vi "flow-builder.ph-dosing.vi"(7 "Proc Name":string, 8 "error in":errorcluster, 9 "Unit Index":i32, 11 "Cluster":T3 {"ORP Dosing"."MIX Limit" format="%d [s]"; "ORP Dosing"."MIX Dose" format="%d [s]"; "PH Dosing"."ACID Limit" format="%d [s]"; "PH Dosing"."BASE Limit" format="%d [s]"; "PH Dosing"."ACID Dose" format="%d [s]"; "PH Dosing"."BASE Dose" format="%d [s]"; "EC Dosing"."BETA2 Limit" format="%d [s]"; "EC Dosing"."ALFA2 Limit" format="%d [s]"; "EC Dosing"."ALFA2 Dose" format="%d [s]"; "EC Dosing"."BETA2 Dose" format="%d [s]"; "EC Dosing"."BETA1 Limit" format="%d [s]"; "EC Dosing"."ALFA1 Limit" format="%d [s]"; "EC Dosing"."ALFA1 Dose" format="%d [s]"; "EC Dosing"."BETA1 Dose" format="%d [s]"; "Main"."DailyActivityHours"."Begin Time" format="ON:    %<%H:%M>T"; "Main"."DailyActivityHours"."End Time" format="OFF:    %<%H:%M>T"; "Main"."WashTimes"."Out" format="Wash out: %d [sec]"; "Main"."WashTimes"."In" format="Wash in: %d [sec]"; "Water Dosing"."Water Limit" format="%d [s]"; "Water Dosing"."Water Dose" format="%d [s]"}) -> (0 "error out":errorcluster, 1 "WillDose?":bool, 2 "status":string, 3 "Flow out":T1[](array[typedef]))   [LabVIEW 2024]
uses:
  controls/UiNutritionPanel.ctl
  controls/UiScheduleTimestamp.ctl
  controls/UiStepBuilder.ctl
  controls/type.step-builder.ctl
  controls/enum-ntr-io-format.ctl
  io.interface.serial.vi
  <vilib>/Utility/error.llb/Clear Errors.vi
  <vilib>/Utility/error.llb/Trim Whitespace One-Sided.vi
  Polymorphics/variantCtrlIo.vi
  globals/globals-engine.vi
  util.environment.vi
  util-address-parser.vi
  util-address-builder.vi
  util.DO.ToString.vi
  Polymorphics/io.command-builder.vi
  Polymorphics/io.command-builder.DO.vi
  Polymorphics/io.command-builder.AI.vi
  Polymorphics/io.command-builder.DI.vi
  io.frame.vi
  io.visa.vi
  io.responseValidator.vi
  Polymorphics/io.command-parser.DI.vi
  Polymorphics/io.command-parser.AI.vi
  step.util.flag-matching.vi
  util.file.record.vi
panel:
  out "Dosing Tabel":cluster{"Dose Time":dbl, "Input":string}[](array[cluster])
  in  "simulator":dbl=3.0
  out "High Range":bool
  out "Low Range":bool
  out "Low Alarm":bool
  out "High Alarm":bool
  # "Water"
  # "EC"
  # "PH"
  # "ORP"
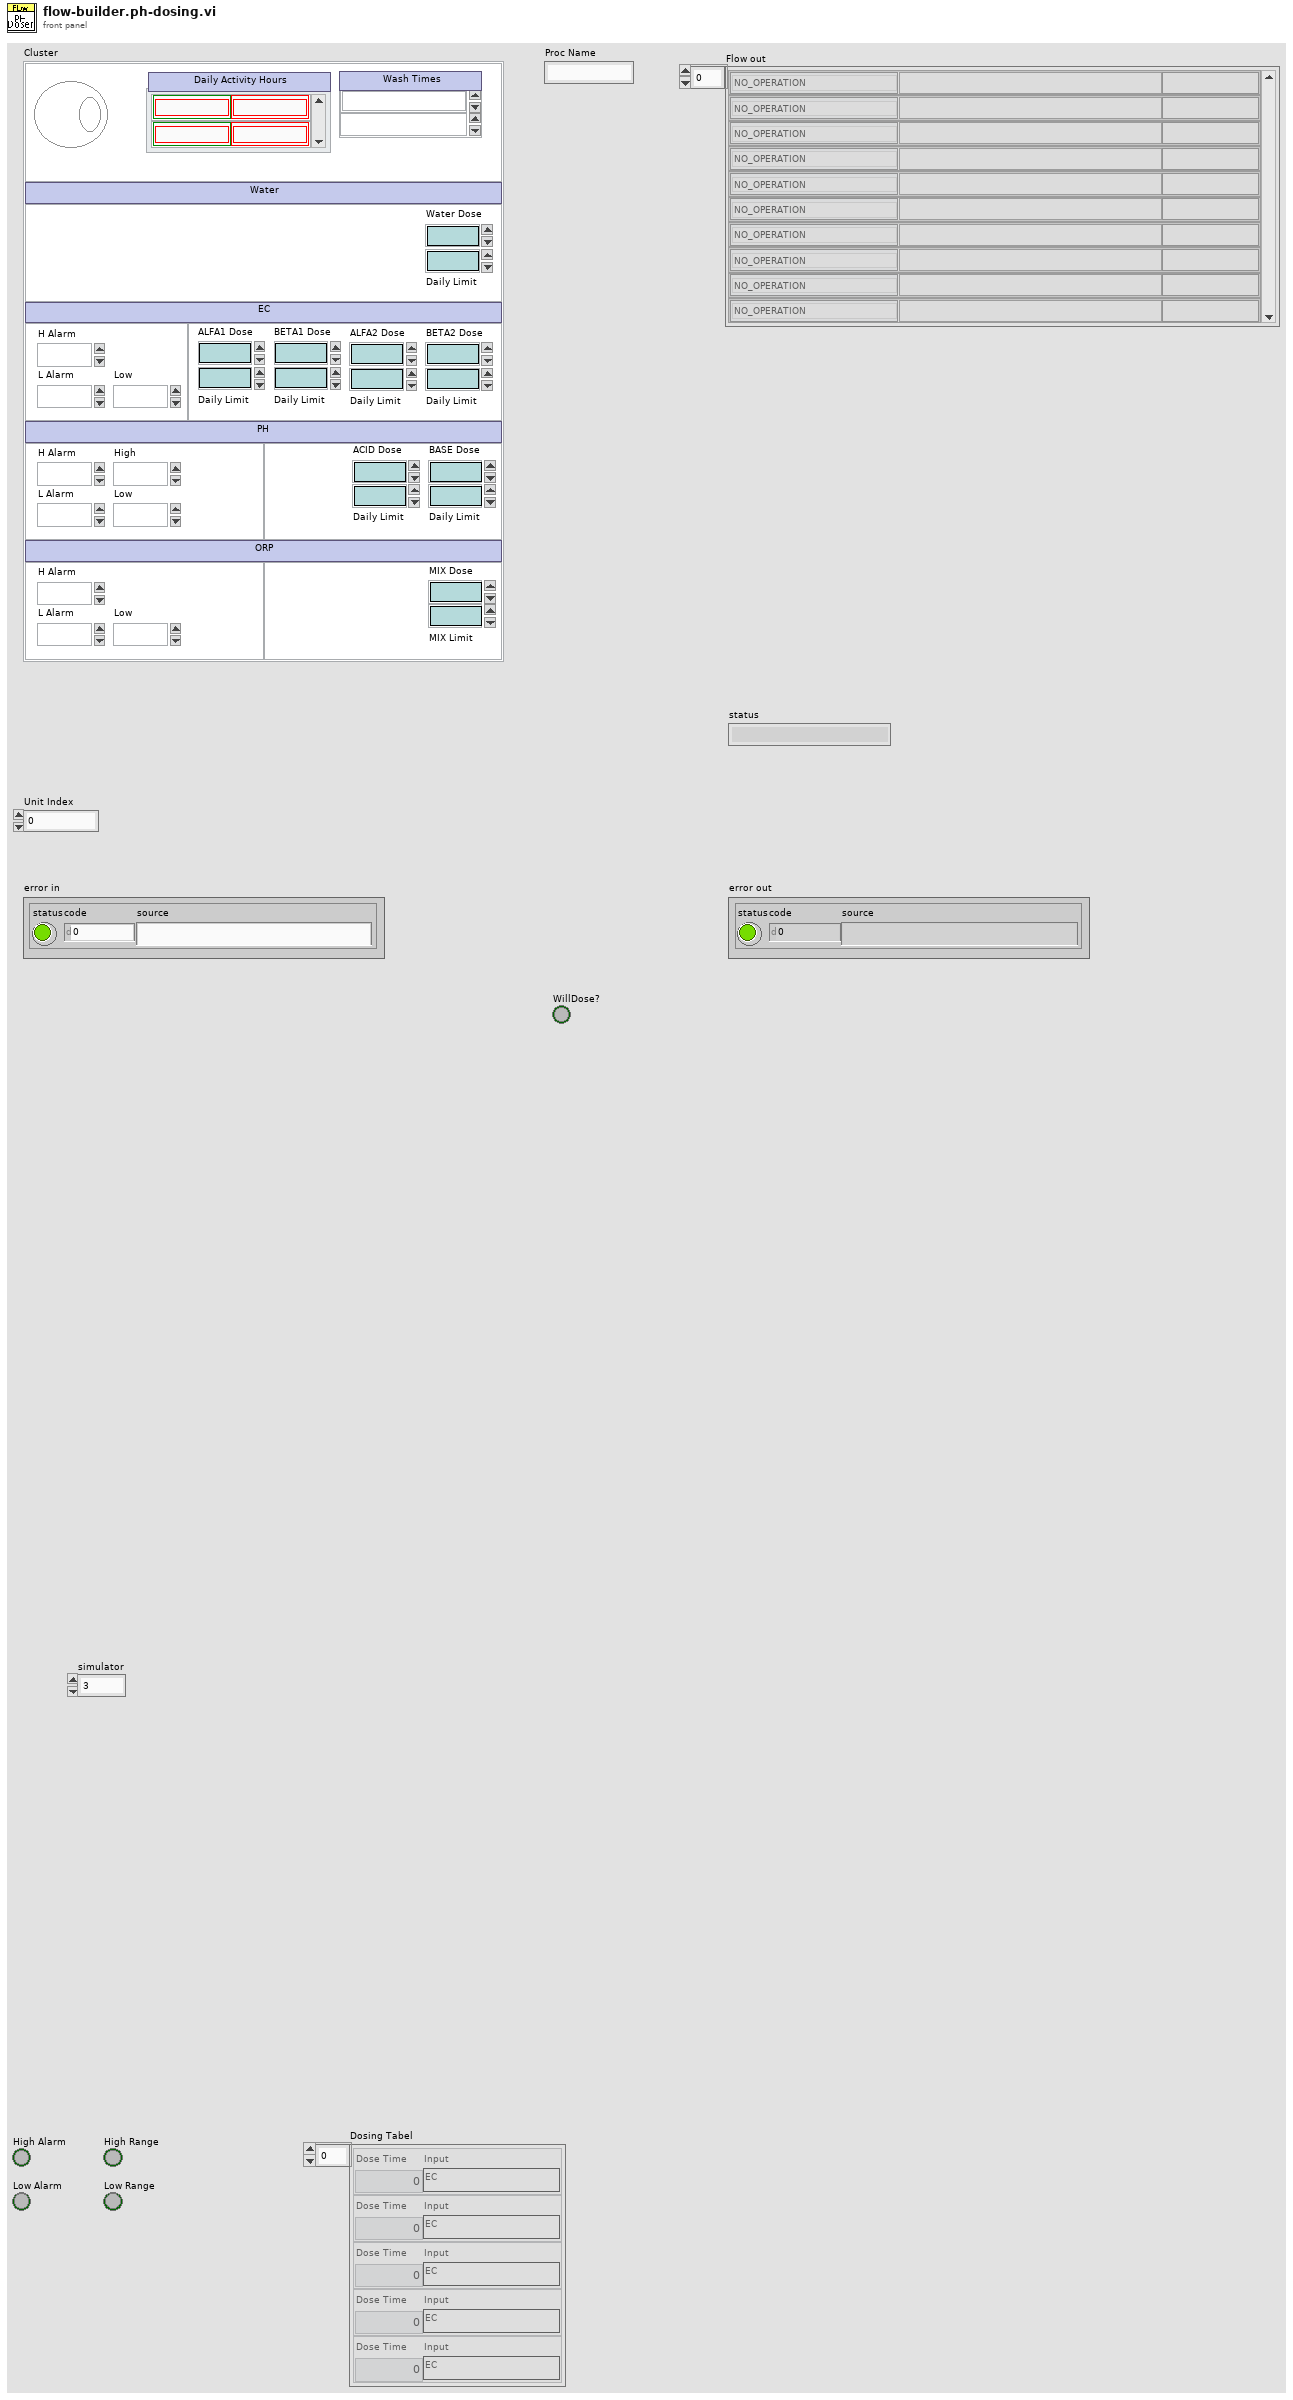
[diagram p1: front panel]
types:
  T1 = typedef "UiStepBuilder.ctl" = cluster{"Step Function":T2, "ParamString":string, "Step Label":string}
  T2 = typedef "type.step-builder.ctl" = enum16{"NO_OPERATION", "DELAY-JUMP", "DELAY", "JUMP", "COMPLETE", "SCHEDULER", "IRR-CHECK", "UNIT-CHECK", "UNIT-SAMPLE", "UNIT-DOSE", "LOG-REPORT", "LOG-MESSAGE", "IO-READ", "IO-READ-MANY", "IO-WRITE", "IO-COMPARE-OUT", "IO-COMPARE-IN", "PROC-START", "PROC-STOP", "PROC-LOAD", "PROC-IS-COMPLETED", "RECORD-MOVE", "GET-RH", "GET-UV", "GET-WD", "GET-WS", "OCS-CHECK", "OCS-RECORD"}
  T3 = typedef "UiNutritionPanel.ctl" = cluster{"Main":cluster{"Enable":bool, "WashTimes":cluster{"In":dbl, "Out":dbl}, "DailyActivityHours":cluster{"Begin Time":T4, "End Time":T4}[]}, "Water Dosing":cluster{"Water Dose":dbl, "Water Limit":dbl}, "EC Ranges":cluster{"H Alarm":dbl, "L Alarm":dbl, "Low":dbl}, "EC Dosing":cluster{"ALFA1 Dose":dbl, "ALFA1 Limit":dbl, "BETA1 Dose":dbl, "BETA1 Limit":dbl, "ALFA2 Dose":dbl, "ALFA2 Limit":dbl, "BETA2 Dose":dbl, "BETA2 Limit":dbl}, "PH Ranges":cluster{"H Alarm":dbl, "L Alarm":dbl, "High":dbl, "Low":dbl}, "PH Dosing":cluster{"ACID Dose":dbl, "ACID Limit":dbl, "BASE Dose":dbl, "BASE Limit":dbl}, "ORP Ranges":cluster{"H Alarm":dbl, "L Alarm":dbl, "Low":dbl}, "ORP Dosing":cluster{"MIX Dose":dbl, "MIX Limit":dbl}}
  T4 = typedef "UiScheduleTimestamp.ctl" = timestamp
  T5 = typedef "enum-ntr-io-format.ctl" = enum16{"UN_VLV%d", "UN_PMP%d", "UN_WL%d", "UN_PH", "UN_EC", "UN_ORP", "UN_WT", "UN_PH2", "UN_ALFA1", "UN_BETA1", "UN_ALFA2", "UN_BETA2", "UN_ACID", "UN_BASE", "UN_WATER", "UN_ORPMIX"}
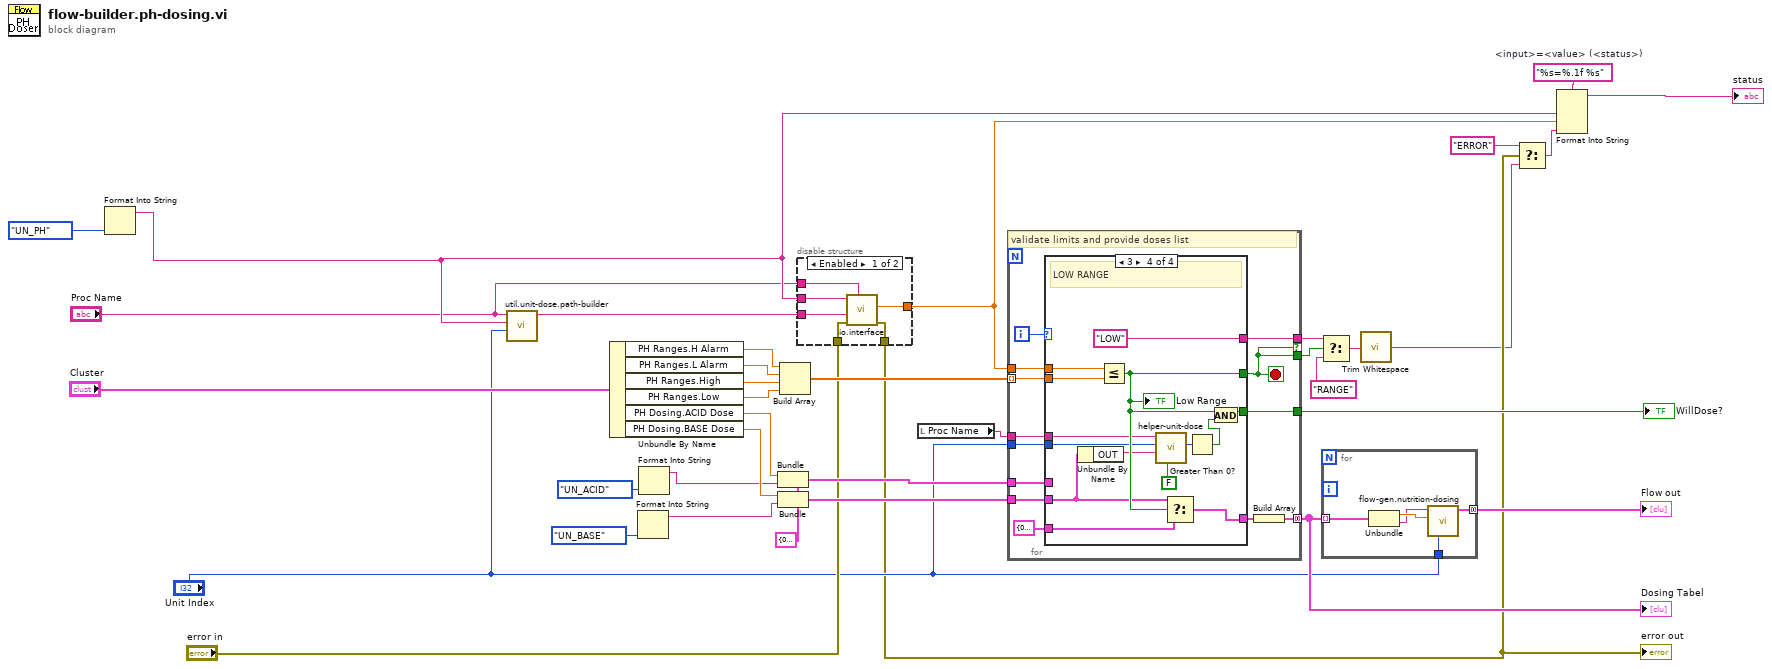
[diagram p0: block diagram]
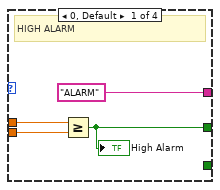
[diagram p2: hidden frame]
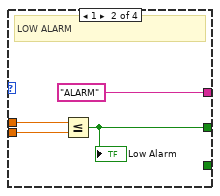
[diagram p3: hidden frame]
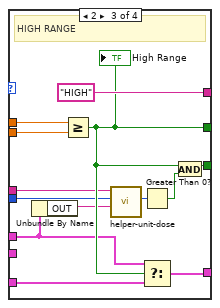
[diagram p4: hidden frame]
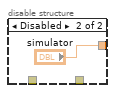
[diagram p5: hidden frame]
diagram:
  w5 = cluster{"ACID Dose":dbl, "OUT":string} {"ACID Dose"=0.0, "OUT"=""} ("cluster")
  w19 = "%s=%.1f %s"  # <input>=<value> (<status>)
  n1 = Format Into String(enum-ntr-io-format."UN_PH") -> (resulting string=w2:string)  [unwired: 3 in, 1 out]
  n2 = call "util.unit-dose.path-builder.vi"("Unit Index"="Unit Index", "Input"=w2, "Proc Name"="Proc Name") -> ("\\NUTRITION\\ORP\\ORP_U1_2024-08-16.*"=w14:string)  [unwired: 8 in]
  n3 = Unbundle By Name("Cluster") -> ("PH Ranges.H Alarm"=w36:dbl, "PH Ranges.L Alarm"=w34:dbl, "PH Ranges.High"=w33:dbl, "PH Ranges.Low"=w32:dbl, "PH Dosing.ACID Dose"=w28:dbl, "PH Dosing.BASE Dose"=w27:dbl)
  n4 = Format Into String(enum-ntr-io-format."UN_BASE") -> (resulting string=w6:string)  [unwired: 3 in, 1 out]
  n5 = Format Into String(enum-ntr-io-format."UN_ACID") -> (resulting string=w7:string)  [unwired: 3 in, 1 out]
  n6 = Bundle(cluster=w5, "ACID Dose"=w28, "OUT"=w7) -> (w26:cluster{"ACID Dose":dbl, "OUT":string})
  n7 = Bundle(cluster=w5, "ACID Dose"=w27, "OUT"=w6) -> (w25:cluster{"ACID Dose":dbl, "OUT":string})
  n8 = Build Array(w36, w34, w33, w32) -> (w35:dbl[])
  n9 = disable-structure shown="Enabled" {
    disable-tunnel: w2 -> [w42 _]
    disable-tunnel: [w41 "simulator"] -> w18
    disable-tunnel: [w40 _] -> w11
    disable-tunnel: "error in" -> [w39 _]
    disable-tunnel: w14 -> [w38 _]
    disable-tunnel: "Proc Name" -> [w37 _]
    frame Enabled {
      n10 = call "io.interface.vi"("Caller"=w37, "error in"=w39, "record filename.* (disabled if empty)"=w38, "IO Name in"=w42) -> ("error out"=w40:errorcluster, "Value out"=w41:dbl)  [unwired: 2 in, 4 out]
    }
    frame Disabled {
    }
  }
  "error out" <- w11
  n11 = local read "Proc Name"() -> (w15:string)
  n12 = for {
    tunnel: w35 -> [w55] mode=indexing
    tunnel: [w54] -> w21 if=w52
    tunnel: w18 -> [w53]
    tunnel: [w52] -> w22
    tunnel: [w49] -> w30 mode=concatenating
    tunnel: w26 -> [w48]
    tunnel: w25 -> [w50]
    tunnel: [w46] -> w16
    tunnel: "Unit Index" -> [w45]
    tunnel: w15 -> [w44]
    i -> [w56]
    stop <- w52 stop-if-true
    # "validate limits and provide doses list"
    n13 = case shown="3" w56 {
      tunnel: w55 -> [w59 w63 w76 w90]
      tunnel: [w57 w61 w72 w86] -> w52
      tunnel: ["ALARM" "ALARM" "HIGH" "LOW"] -> w54
      tunnel: w53 -> [w58 w62 w75 w89]
      tunnel: [_ _ w74 w88] -> w51
      tunnel: w50 -> [_ _ _ w83]
      tunnel: w48 -> [_ _ w65 _]
      tunnel: cluster{"BETA-2":dbl, "I/O":string} {"BETA-2"=0.0, "I/O"=""} ("f") -> [_ _ w73 w87]
      tunnel: [_ _ w67 w80] -> w46
      tunnel: w45 -> [_ _ w68 w81]
      tunnel: w44 -> [_ _ w69 w78]
      frame 0, Default {
        # "HIGH ALARM"
        n14 = Greater Or Equal?(x=w58, y=w59) -> (x >= y?=w57:bool)
        "High Alarm" <- w57
      }
      frame 1 {
        # "LOW ALARM"
        n15 = Less Or Equal?(x=w62, y=w63) -> (x <= y?=w61:bool)
        "Low Alarm" <- w61
      }
      frame 2 {
        # "HIGH RANGE"
        n16 = Unbundle By Name(w65) -> ("OUT"=w70:string)
        n17 = Greater Or Equal?(x=w75, y=w76) -> (x >= y?=w72:bool)
        "High Range" <- w72
        n18 = call "helper-unit-dose.vi"("output"=w70, "Unit Index"=w68, "Proc Name"=w69) -> ("Actual Dose in Seconds"=w71:i32)  [unwired: 6 in, 2 out]
        n19 = Greater Than 0?(x=w71) -> (x > 0?=w66:bool)
        n20 = Select(t=w65, s=w72, f=w73) -> (s? t:f=w74:cluster{"BETA-2":dbl, "I/O":string})
        n21 = And(x=w72, y=w66) -> (x .and. y?=w67:bool)
      }
      frame 3 {
        # "LOW RANGE"
        n22 = Unbundle By Name(w83) -> ("OUT"=w82:string)
        n23 = Less Or Equal?(x=w89, y=w90) -> (x <= y?=w86:bool)
        "Low Range" <- w86
        n24 = call "helper-unit-dose.vi"("Auto Update Limit Record? (T)"=FALSE ("(F)ReadOnly/(T)Auto Update"), "output"=w82, "Unit Index"=w81, "Proc Name"=w78) -> ("Actual Dose in Seconds"=w84:i32)  [unwired: 5 in, 2 out]
        n25 = Select(t=w83, s=w86, f=w87) -> (s? t:f=w88:cluster{"BETA-2":dbl, "I/O":string})
        n26 = Greater Than 0?(x=w84) -> (x > 0?=w79:bool)
        n27 = And(x=w86, y=w79) -> (x .and. y?=w80:bool)
      }
    }
    n28 = Build Array(w51) -> (w49:cluster{"BETA-2":dbl, "I/O":string}[])
  }
  "Dosing Tabel" <- w30
  "WillDose?" <- w16
  n29 = Select(t=w21, s=w22, f="RANGE") -> (s? t:f=w17:string)
  n30 = for {
    tunnel: [w96] -> w29 mode=concatenating
    tunnel: w30 -> [w95] mode=indexing
    tunnel: "Unit Index" -> [w92]
    n31 = Unbundle(w95) -> ("BETA-2"=w94:dbl, "I/O"=w93:string)
    n32 = call "flow-gen.nutrition-dosing.vi"("Unit Index"=w92, "Dosing Time"=w94, "IO Name"=w93) -> ("Flow"=w96:T1[])  [unwired: 7 in, 1 out]
  }
  "Flow out" <- w29
  n33 = call <vilib>:"Trim Whitespace.vi"("string"=w17) -> ("trimmed string"=w10:string)  [unwired: 1 in]
  n34 = Select(t="ERROR", s=w11, f=w10) -> (s? t:f=w9:string)
  n35 = Format Into String(format string=w19, w2, w18, w9) -> (resulting string=→"status":string)  [unwired: 2 in, 1 out]
